vi "AssertControlValueByName.vi"(0 "VI Reference In":refnum<vi>, 2 "delimiter (Tab)":string, 5 "Control Name":string, 11 "error in":errorcluster) -> (4 "VI Reference Out":refnum<vi>, 6 "Value":variant, 15 "error out":errorcluster)   [LabVIEW 2016]
doc: "This VI sets the value of top level controls in other VI"
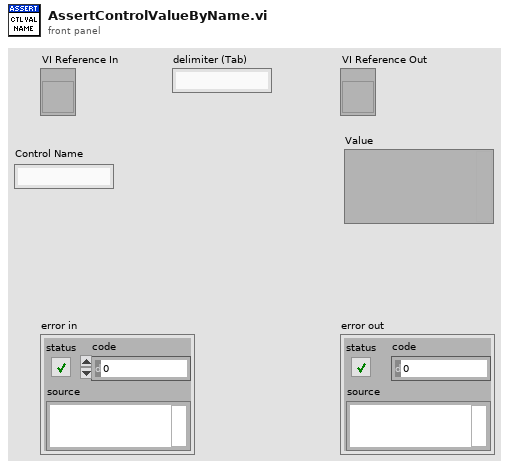
[diagram p1: front panel]
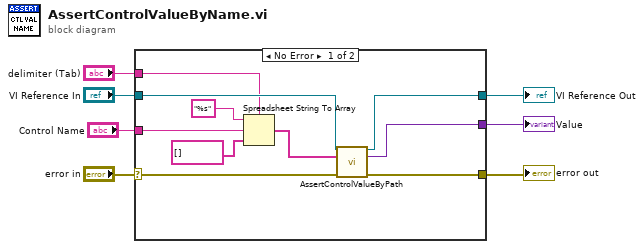
[diagram p0: block diagram]
diagram:
  n1 = case shown="No Error" "error in" {
    selector: "error in" -> [w16 w19]
    tunnel: "Control Name" -> [w12 _]
    tunnel: "VI Reference In" -> [w17 w18]
    tunnel: [w14 w18] -> w4
    tunnel: [w15 w19] -> w3
    tunnel: [w13 _] -> w2
    tunnel: "delimiter (Tab)" -> [w8 _]
    frame No Error {
      n2 = Spreadsheet String To Array(delimiter (Tab)=w8, format string="%s", spreadsheet string=w12, array type (2D Dbl)=string[] []) -> (array=w10:string[])
      n3 = call "AssertControlValueByPath.vi"("VI Reference In"=w17, "Control Path"=w10, "error in"=w16) -> ("VI Reference Out"=w14:refnum<vi>, "Value"=w13:variant, "error out"=w15:errorcluster)  [unwired: 10 in]
    }
    frame Error {
    }
  }
  "error out" <- w3
  "VI Reference Out" <- w4
  "Value" <- w2
